vi "Get VI Information.vi"() -> ()   [LabVIEW 2017]
doc: "Retrieves the information from the active VI"
uses:
  Connector Pane Patterns.ctl
panel:
  in  "Tab Control":enum32{"General", "Documentation", "Execution"}(tab)
  out "ConPane Pattern":T1=3
  out "Icon":picture
  out "VI Revision":u32
  out "Hist.Text":string
  out "Source Version":string
  out "SeparateCompiledCode":bool caption="Compiled code separated from source file"
  out "Path":path
  out "Name":string
  in  "Bookmarks":i32(listbox)
  out "VI Help.Doc":string
  out "VI Help.Tag":string
  out "Description":string
  out "SuspOnCall":bool
  out "Def Err Handling":bool
  out "RunOnOpen":bool
  out "Reentrancy Type":T2(ring)
  out "Priority":T3(ring)
  out "Preferred Exec System":T4(ring)
  out "Is Reentrant":bool
  out "Allow Debugging":bool
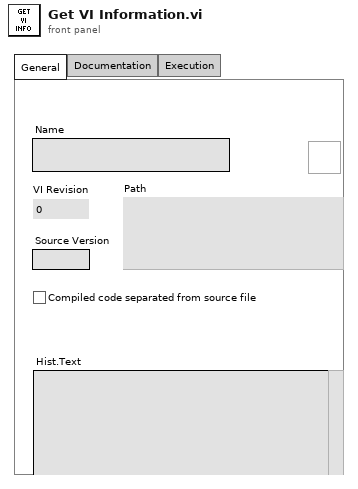
[diagram p1: front panel]
types:
  T1 = typedef "Connector Pane Patterns.ctl" = i32
  T2 = enum16{"Share clones between instances", "Preallocate clone for each instance"}
  T3 = enum32{"invalid priority", "background priority", "normal priority", "above normal priority", "high priority", "time critical priority", "subroutine"}
  T4 = enum32{"invalid execution system", "user interface", "standard", "instrument i/o", "data acquisition", "other 1", "other 2", "same as caller"}
  T5 = cluster{"VI Name":string, "VI Path":path, "VI Revision":u32, "VI History":string, "CompileCodeSeparated":bool, "VI Version":cluster{"VI Version":string, "VI Vers":u32, "VI Editor Version":string, "VI Editor Vers":u32}, "ConPane Pattern":T1, "Icon Image":picture}
  T6 = cluster{"VI Description":string, "VI Help.Tag":string, "VI Help.Doc":string}
  T7 = cluster{"AllowDebugging":bool, "IsReentrant":bool, "ReentrancyType":enum16{"Share clones between instances", "Preallocate clone for each instance"}, "PrefSys":enum32{"invalid execution system", "user interface", "standard", "instrument i/o", "data acquisition", "other 1", "other 2", "same as caller"}, "riority":enum32{"invalid priority", "background priority", "normal priority", "above normal priority", "high priority", "time critical priority", "subroutine"}, "RunOnOpen":bool, "Def Err Handling":bool, "SuspOnCall":bool}
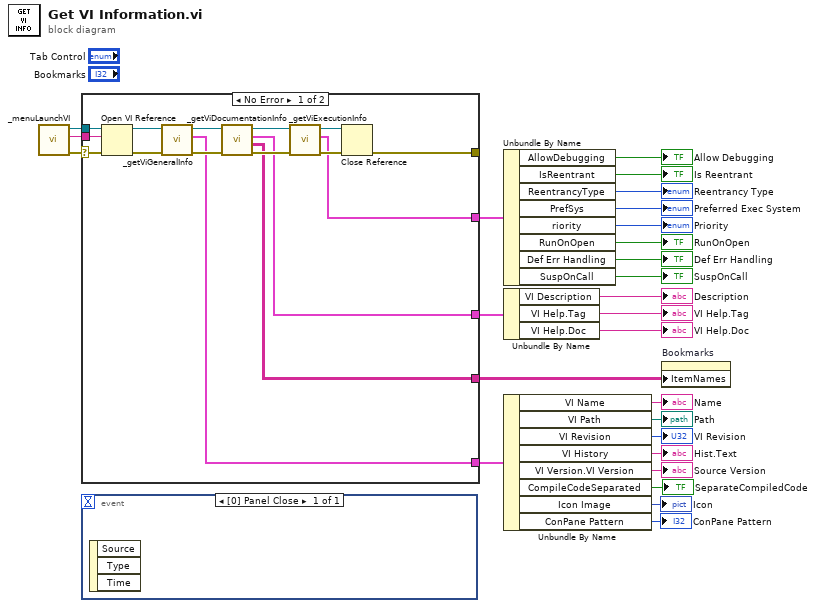
[diagram p0: block diagram]
diagram:
  n1 = call "_menuLaunchVI.vi"() -> ("error out"=w26:errorcluster, "Menu Launch:VI"=w25:string, "Menu Launch:App"=w24:refnum<vi>)  [unwired: 9 in]
  n2 = case shown="No Error" w26 {
    selector: w26 -> [w42 w43]
    tunnel: w25 -> [w41 _]
    tunnel: w24 -> [w40 _]
    tunnel: [w39 w43] -> _
    tunnel: [w30 _] -> w23
    tunnel: [w27 _] -> w1
    tunnel: [w29 _] -> w17
    tunnel: [w28 _] -> w13
    frame No Error {
      n3 = Open VI Reference(application reference (local)=w40, vi path=w41, error in (no error)=w42) -> (vi reference=w38:refnum<vi>, error out=w37:errorcluster)  [unwired: 3 in]
      n4 = call "_getViGeneralInfo.vi"("error in (no error)"=w37, "VI in"=w38) -> ("error out"=w35:errorcluster, "VI General Info"=w30:T5, "VI out"=w36:refnum<vi>)  [unwired: 7 in]
      n5 = call "_getViDocumentationInfo.vi"("error in (no error)"=w35, "VI in"=w36) -> ("error out"=w33:errorcluster, "Bookmarks"=w27:string[][], "VI Documentation Info"=w29:T6, "VI out"=w34:refnum<vi>)  [unwired: 6 in]
      n6 = call "_getViExecutionInfo.vi"("error in (no error)"=w33, "VI in"=w34) -> ("error out"=w32:errorcluster, "VI Execution Info"=w28:T7, "VI out"=w31:refnum<vi>)  [unwired: 7 in]
      n7 = Close Reference(reference=w31, error in (no error)=w32) -> (error out=w39:errorcluster)
    }
    frame Error {
    }
  }
  n8 = event shown="[0] Panel Close" {
    selector: _ -> [_]
    dyn-events: _ -> [_]
    timeout: _ -> [_]
    event Panel Close {
      n9 = event-data() -> ()  [unwired: 1 in, 3 out]
    }
  }
  n10 = Unbundle By Name(w13) -> ("AllowDebugging"=→"Allow Debugging":bool, "IsReentrant"=→"Is Reentrant":bool, "ReentrancyType"=→"Reentrancy Type":T2, "PrefSys"=→"Preferred Exec System":T4, "riority"=→"Priority":T3, "RunOnOpen"=→"RunOnOpen":bool, "Def Err Handling"=→"Def Err Handling":bool, "SuspOnCall"=→"SuspOnCall":bool)
  n11 = Unbundle By Name(w17) -> ("VI Description"=→"Description":string, "VI Help.Tag"=→"VI Help.Tag":string, "VI Help.Doc"=→"VI Help.Doc":string)
  n12 = Unbundle By Name(w23) -> ("VI Name"=→"Name":string, "VI Path"=→"Path":path, "VI Revision"=→"VI Revision":u32, "VI History"=→"Hist.Text":string, "VI Version.VI Version"=→"Source Version":string, "CompileCodeSeparated"=→"SeparateCompiledCode":bool, "Icon Image"=→"Icon":picture, "ConPane Pattern"=→"ConPane Pattern":T1)
  n13 = property on="Bookmarks" class="MCListbox (strict)"("ItemNames"=w1) -> ()  [unwired: 2 in, 2 out]
